vi "set.FieldSpecs.vi"(8 "error in (no error)":errorcluster, 10 "Field Specs":T1[](array[typedef])=[{"Length", "Offset"=0, "Length"=1, "FieldType"=enum."Binary"}, {"MessageType", "Offset"=1, "Length"=1, "FieldType"=enum."Value"}, {"Time Offset", "Offset"=2, "Length"=4, "FieldType"=enum."Binary"}, {"Order Id", "Offset"=6, "Length"=8, "FieldType"=enum."Binary"}, {"Side Indicator", "Offset"=14, "Length"=1, "FieldType"=enum."Alphanumeric"}, {"Quantity", "Offset"=15, "Length"=4, "FieldType"=enum."Binary"}, {"Symbol", "Offset"=19, "Length"=6, "FieldType"=enum."PrintableAscii"}, {"Price", "Offset"=25, "Length"=8, "FieldType"=enum."BinaryLongPrice"}, {"Add Flags", "Offset"=33, "Length"=1, "FieldType"=enum."BitField"}], 11 "PitchMessage in":refnum<class "PitchMessage.lvclass">) -> (0 "error out":errorcluster, 3 "PitchMessage out":refnum<class "PitchMessage.lvclass">)   [LabVIEW 2022 SP3, in "PitchMessage.lvclass"]
uses:
  PitchMessage.lvclass
  FieldSpec.ctl
  PitchMessage.lvclass/PitchMessage.ctl
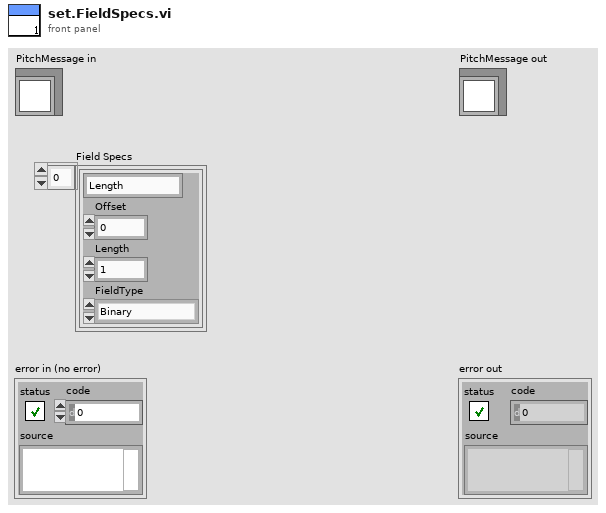
[diagram p1: front panel]
types:
  T1 = typedef "FieldSpec.ctl" = cluster{string, "Offset":i32, "Length":i32, "FieldType":enum16{"Alphanumeric", "Binary", "BinaryLongPrice", "BinaryShortPrice", "BitField", "PrintableAscii", "Value"}}
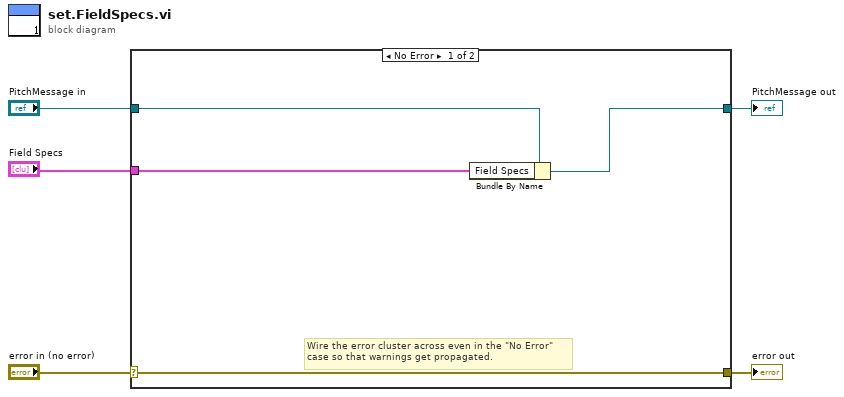
[diagram p0: block diagram]
diagram:
  n1 = case shown="No Error" "error in (no error)" {
    selector: "error in (no error)" -> [w9 w11]
    tunnel: [w9 w11] -> w4
    tunnel: [w6 w10] -> w2
    tunnel: "PitchMessage in" -> [w7 w10]
    tunnel: "Field Specs" -> [w8 _]
    frame No Error {
      # "Wire the error cluster across even in the \"No Error\"\ncase so that warnings get propagated."
      n2 = Bundle By Name(cluster=w7, "Field Specs"=w8) -> (w6:refnum<class "PitchMessage.lvclass">)
    }
    frame Error {
    }
  }
  "error out" <- w4
  "PitchMessage out" <- w2
